vi "NMR13.vi"() -> ()   [LabVIEW 2013]
uses:
  <vilib>/Analysis/NI_AALBase.lvlib
panel:
  in  "AutoBaseline":bool=TRUE
  out "RF OK":bool=TRUE
  out "Peak area (V-MHz)":sgl=0.08843879 format="%.3f"
  in  "Gauss Fit":bool
  out "NMR Graph + Fit":cluster{cluster{dbl, "Numeric":dbl}[]}[](graph)=[{[{212.6, "Numeric"=0.037403535286502254}, {212.608, "Numeric"=0.009076660286615634}, {212.61599999999999, "Numeric"=0.027280678255148183}, {212.624, "Numeric"=0.041539514974009595}, {212.632, "Numeric"=0.042392721224115915}, {212.64, "Numeric"=0.02815572669266192}, {212.648, "Numeric"=0.028369547005266005}, {212.656, "Numeric"=0.02612744388036531}, {212.664, "Numeric"=0.028228733723923927}, {212.672, "Numeric"=0.03396540872402104}, {212.68, "Numeric"=0.032192449349113195}, {212.688, "Numeric"=0.03708221888018509}, {212.696, "Numeric"=0.032277295442774745}, {212.704, "Numeric"=0.033878753255359884}, {212.712, "Numeric"=0.03956725638019448}, {212.72, "Numeric"=0.02444046106777714}, {212.728, "Numeric"=0.03311506653637314}, {212.736, "Numeric"=0.03391382669270321}, {212.744, "Numeric"=0.028289378255278386}, {212.752, "Numeric"=0.03139064700513733}, {212.76, "Numeric"=0.034697125130210116}, {212.768, "Numeric"=0.022986644661528388}, {212.776, "Numeric"=0.0246283462239002}, {212.784, "Numeric"=0.020225257161465893}, {212.792, "Numeric"=0.019823764192777038}, {212.79999999999998, "Numeric"=0.024168496223911762}, {212.808, "Numeric"=0.019062675911470317}, {212.816, "Numeric"=0.019752885286524247}, {212.82399999999998, "Numeric"=0.015045276692672138}, {212.832, "Numeric"=0.0044881899739736}, {212.84, "Numeric"=0.013533285286520313}, {212.84799999999998, "Numeric"=0.028093648567681206}, {212.856, "Numeric"=0.011194182161475441}, {212.864, "Numeric"=0.04047160481776502}, {212.87199999999999, "Numeric"=0.029683240755188967}, {212.88, "Numeric"=0.03155125794272601}, {212.888, "Numeric"=0.01863425013025849}, {212.896, "Numeric"=0.03868612356769546}, {212.904, "Numeric"=0.05375521809897532}, {212.912, "Numeric"=0.05373411184900062}, {212.92, "Numeric"=0.0648435079427006}, {212.928, "Numeric"=0.08718106263022335}, {212.936, "Numeric"=0.10025117044274146}, {212.944, "Numeric"=0.1585216048177045}, {212.952, "Numeric"=0.2650075024739701}, {212.96, "Numeric"=0.46508239856773104}, {212.968, "Numeric"=0.8254088907552071}, {212.976, "Numeric"=1.0513580727864655}, {212.984, "Numeric"=0.8573220345052025}, {212.992, "Numeric"=0.6793237251302083}, {213.0, "Numeric"=0.6370530860677096}, {213.008, "Numeric"=0.6190965430989597}, {213.016, "Numeric"=0.49919677200520834}, {213.024, "Numeric"=0.44351588216145243}, {213.032, "Numeric"=0.4586334634114655}, {213.04, "Numeric"=0.47208857825520706}, {213.048, "Numeric"=0.434772339973944}, {213.056, "Numeric"=0.4489796704427201}, {213.064, "Numeric"=0.46391711263020446}, {213.072, "Numeric"=0.3840036118489343}, {213.08, "Numeric"=0.27875821106772336}, {213.088, "Numeric"=0.2001462423177006}, {213.096, "Numeric"=0.12634153372392326}, {213.104, "Numeric"=0.10264437825522532}, {213.112, "Numeric"=0.09343465872394546}, {213.12, "Numeric"=0.0575136446614109}, {213.12800000000001, "Numeric"=0.03758153138022602}, {213.136, "Numeric"=0.021797498567688922}, {213.144, "Numeric"=-0.00047077799485278904}, {213.15200000000002, "Numeric"=-0.0034786694010245367}, {213.16, "Numeric"=0.020452047005181218}, {213.168, "Numeric"=0.045967367317632346}, {213.17600000000002, "Numeric"=0.0187704165364736}, {213.184, "Numeric"=-0.008209117838577862}, {213.192, "Numeric"=-0.014756392057383827}, {213.2, "Numeric"=-0.02673810533852966}, {213.208, "Numeric"=-0.04046773424483824}, {213.216, "Numeric"=-0.046704556119901375}, {213.224, "Numeric"=-0.05625179361978411}, {213.232, "Numeric"=-0.04296198580734978}, {213.24, "Numeric"=-0.05743327721347158}, {213.248, "Numeric"=-0.06834242565103987}, {213.256, "Numeric"=-0.06423923580736263}, {213.264, "Numeric"=-0.06864665690097155}, {213.272, "Numeric"=-0.07023656393229688}, {213.28, "Numeric"=-0.056496749869876794}, {213.288, "Numeric"=-0.045896452994722836}, {213.296, "Numeric"=-0.05285217721355545}, {213.304, "Numeric"=-0.03777652018239258}, {213.312, "Numeric"=-0.024912645963475255}, {213.32, "Numeric"=-0.030617976432314953}, {213.328, "Numeric"=-0.02721917174490912}, {213.336, "Numeric"=-0.029767501432229004}, {213.344, "Numeric"=-0.01918337565107603}, {213.352, "Numeric"=-0.013301267057427346}, {213.36, "Numeric"=-0.01544148815098395}, {213.368, "Numeric"=-0.004363804557338036}, {213.376, "Numeric"=0.001474752473802965}, {213.38400000000001, "Numeric"=0.00859273763025964}, {213.392, "Numeric"=0.012363686067648316}, {213.4, "Numeric"=0.002082031380032434}]}]
  in  "Amp of Q curve":dbl=14.8 format="%_3f"
  in  "Subtract Q curve":bool=TRUE
  in  "Adjust Tune":bool
  out "IF Offset":dbl(graph)=3.0267583007812493
  out "Pedestal Difference":dbl(graph)=-0.055571065625063976
  out "# Good Spectra":i32=99
  in  "Quality cuts":bool=TRUE
  out "Pedestal OK":bool=TRUE
  out "Sweep #":i32=100
  out "1st Sweep":bool
  out "ADC volts OK":bool=TRUE
  out "Peak Height Distribution":cluster{"Y":dbl[], "Y":dbl[]}[](graph)=[{"Y"=[1.0290775755533925, 1.0294921670247466, 1.0299067584961008, 1.030321349967455, 1.030735941438809, 1.0311505329101633, 1.0315651243815174, 1.0319797158528716, 1.0323943073242259, 1.03280889879558, 1.0332234902669342, 1.0336380817382884, 1.0340526732096424, 1.0344672646809967, 1.0348818561523507, 1.035296447623705, 1.0357110390950592, 1.0361256305664133, 1.0365402220377675, 1.0369548135091216, 1.0373694049804758, 1.03778399645183, 1.038198587923184, 1.0386131793945383, 1.0390277708658924, 1.0394423623372466, 1.0398569538086009, 1.040271545279955, 1.0406861367513092, 1.0411007282226632, 1.0415153196940174, 1.0419299111653717, 1.0423445026367257, 1.04275909410808, 1.0431736855794342, 1.0435882770507883, 1.0440028685221425, 1.0444174599934966, 1.0448320514648508, 1.045246642936205, 1.045661234407559, 1.0460758258789133, 1.0464904173502674, 1.0469050088216216, 1.0473196002929759, 1.04773419176433, 1.0481487832356842, 1.0485633747070382, 1.0489779661783925, 1.0493925576497467, 1.0498071491211007, 1.050221740592455, 1.0506363320638092, 1.0510509235351633, 1.0514655150065175, 1.0518801064778716, 1.0522946979492258, 1.05270928942058, 1.053123880891934, 1.0535384723632883, 1.0539530638346424, 1.0543676553059966, 1.0547822467773509, 1.055196838248705, 1.0556114297200592, 1.0560260211914132, 1.0564406126627675, 1.0568552041341217, 1.0572697956054757, 1.05768438707683, 1.058098978548184, 1.0585135700195383, 1.0589281614908925, 1.0593427529622466, 1.0597573444336008, 1.060171935904955, 1.060586527376309, 1.0610011188476633, 1.0614157103190174, 1.0618303017903716, 1.0622448932617259, 1.06265948473308, 1.0630740762044342, 1.0634886676757882, 1.0639032591471425, 1.0643178506184967, 1.0647324420898507, 1.065147033561205, 1.065561625032559, 1.0659762165039133, 1.0663908079752675, 1.0668053994466216, 1.0672199909179758, 1.06763458238933, 1.068049173860684, 1.0684637653320384, 1.0688783568033924, 1.0692929482747466, 1.0697075397461009, 1.070122131217455], "Y"=[1.0, 0.0, 0.0, 0.0, 0.0, 0.0, 0.0, 0.0, 0.0, 0.0, 0.0, 0.0, 0.0, 1.0, 0.0, 0.0, 0.0, 0.0, 0.0, 1.0, 1.0, 0.0, 0.0, 2.0, 0.0, 0.0, 0.0, 2.0, 0.0, 2.0, 0.0, 2.0, 0.0, 3.0, 0.0, 4.0, 2.0, 1.0, 1.0, 2.0, 1.0, 1.0, 2.0, 0.0, 0.0, 2.0, 0.0, 1.0, 1.0, 1.0, 1.0, 2.0, 1.0, 3.0, 2.0, 1.0, 0.0, 4.0, 2.0, 1.0, 3.0, 1.0, 1.0, 4.0, 3.0, 3.0, 2.0, 0.0, 2.0, 0.0, 2.0, 0.0, 1.0, 2.0, 1.0, 1.0, 2.0, 3.0, 1.0, 1.0, 0.0, 1.0, 0.0, 1.0, 2.0, 0.0, 0.0, 1.0, 1.0, 2.0, 1.0, 1.0, 2.0, 0.0, 0.0, 1.0, 0.0, 1.0, 0.0, 1.0]}]
  in  "# of Sweeps":i32=100
  out "Std Dev (V)":dbl=0.008821657917615048 format="%_2g"
  out "Peak mean (V)":dbl=1.0528182762205458 format="%_4g"
  out "Peak Height":dbl(graph)=1.0513580727864655
  in  "Raw Data":bool=TRUE
  in  "Tank RF ON":bool=TRUE
  in  "IF Atten (dB)":i8 min=0 max=35 step=5
  in  "IFoffset (V)":dbl=3.026265771484374 min=0.0 max=3000.0 step=0.001 format="%.3f"
  in  "Tune  (V)":dbl=1.9290000000000005 min=0.0 max=5.0 step=0.001 format="%.3f"
  in  "Hi / Lo Gain":bool
  out "Voltage Array":sgl[](array[numeric])=[2.0380492, 1.9150025, 1.8403809, 1.7637085, 1.675525, 1.5741456, 1.4891113, 1.4035156, 1.3241577, 1.2503296, 1.1708863, 1.1, 1.0213134, 0.95092773, 0.8865234, 0.8031982, 0.7455689, 0.681958, 0.61381835, 0.55629885, 0.50087893, 0.43233642, 0.37904054, 0.32159424, 0.27004394, 0.22513428, 0.17266846, 0.12789306, 0.07961426, 0.027380371, -0.0033569336, -0.026684571, -0.07957764, -0.08439942, -0.12739258, -0.15583496, -0.19716796, -0.20363769, -0.2131958, -0.23594971, -0.24567871, -0.24228516, -0.24626465, -0.20314941, -0.10992432, 0.07878418, 0.42963868, 0.64801025, 0.448291, 0.2665039, 0.22233887, 0.20438233, 0.08637695, 0.034484863, 0.055285644, 0.07631836, 0.04847412, 0.07404785, 0.10224609, 0.037487794, -0.050708007, -0.11037598, -0.16334228, -0.16430664, -0.14888915, -0.15828857, -0.14980468, -0.13527831, -0.1253418, -0.094250485, -0.034326173, 0.029077148, 0.041662596, 0.056359865, 0.09338379, 0.12686768, 0.16049805, 0.20351562, 0.24511719, 0.31145018, 0.3519165, 0.39783937, 0.46066895, 0.5168823, 0.5778076, 0.65595704, 0.73286134, 0.794104, 0.87927246, 0.96412355, 1.0322998, 1.1114746, 1.1865966, 1.2767456, 1.3640869, 1.4453003, 1.541626, 1.634607, 1.7307618, 1.8254639, 1.9080079] format="%.4f"
  in  "Invert Polarity":bool=TRUE
  out "Pedestal Diff (V)":sgl=-0.055571064 format="%.3f"
  out "Peak amp (V)":sgl=1.0513581 format="%.3f"
  in  "Save Data to File":bool
  in  "RF Level (dBm)":dbl min=-10.0 max=1.0 step=0.1 format="%.2f"
  out "SMT error out":errorcluster
  out "Sample RMS (V)":dbl=0.013290809562570826 format="%.4f"
  in  "# Sample/step":i32=100 min=1 max=1000 step=100
  in  "ADC Rate (Hz)":i32=10000 min=1 max=20000 step=1000
  in  "ADC Range":i32(ring)=1 items=["+- 10 V"=1, "+- 2.5 V"=3]
  in  "Step Width (MHz)":dbl=0.008 min=0.0 max=1000.0 step=0.0005 format="%.4f"
  in  "Freq Span (MHz)":dbl=0.8 min=0.0 max=3000.0 step=0.1 format="%.3f"
  in  "Center Freq (MHz)":dbl=213.0 min=0.005 max=6000.0 step=0.1 format="%.3f"
  in  "Sweep Mode":u16(ring)=3 items=["Off", "Single", "Auto", "Step"]
  in  "GPIB Addr (28)":refnum<visa-resource-name>="GPIB0::28::INSTR"
  # "Settings"
  # "E1039 Prototype NMR Control Panel"
  # "D\nA\nC"
  # "R\nF\n\nG\ne\nn\ne\nr\na\nt\no\nr"
  # "A\nD\nC"
  # "D\na\nt\na"
  # "I\n/\nO"
  # "Results"
  # "A\nv\ne\nr\na\ng\ne"
  # "S\nw\ne\ne\np"
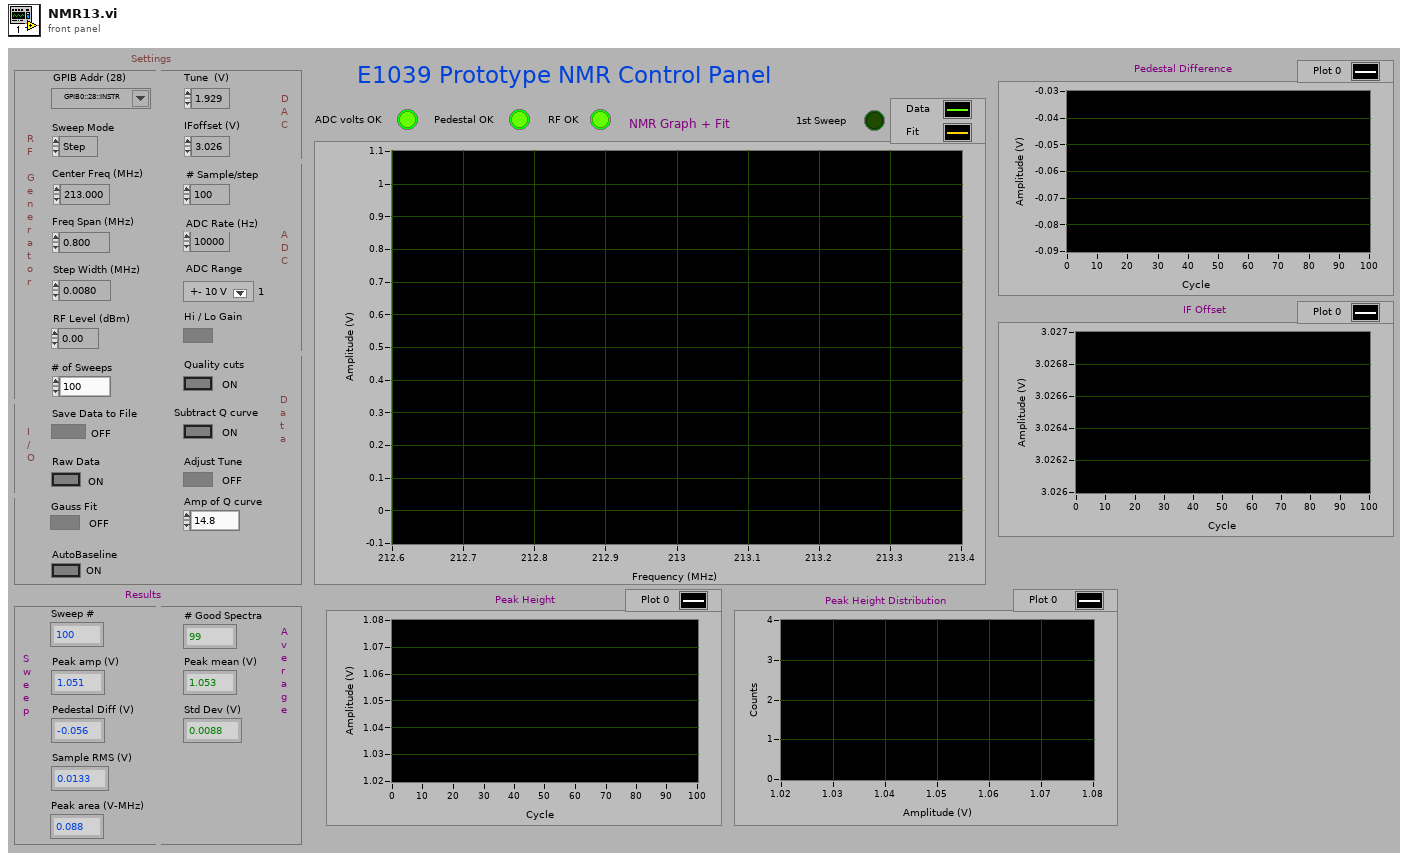
[diagram p1: front panel]
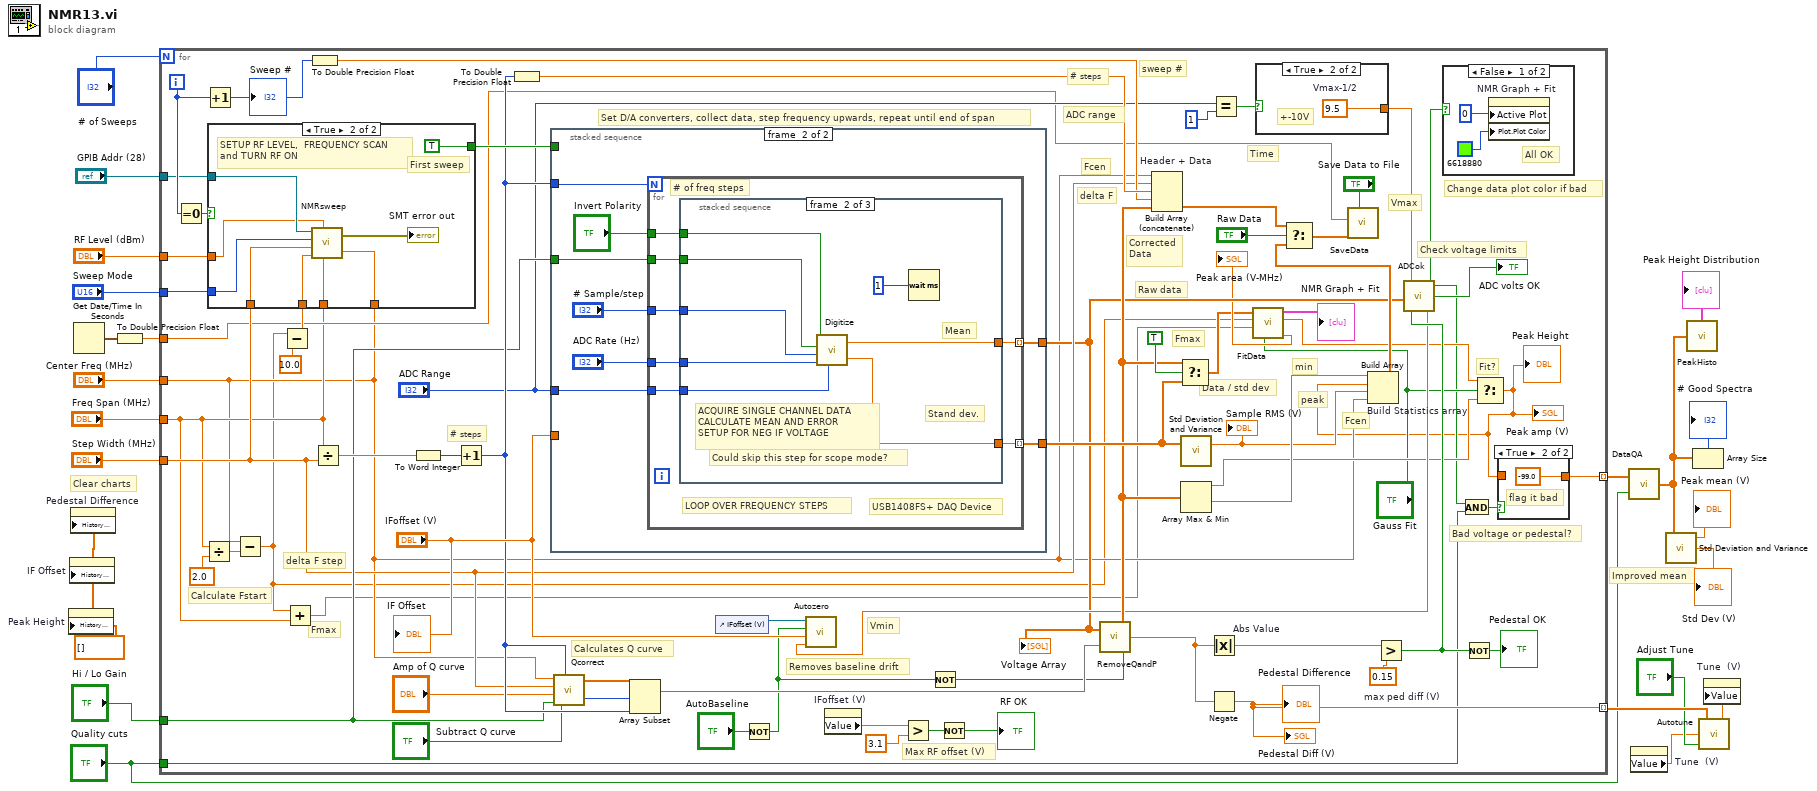
[diagram p0: block diagram]
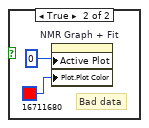
[diagram p2: hidden frame]
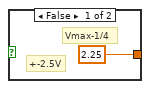
[diagram p3: hidden frame]
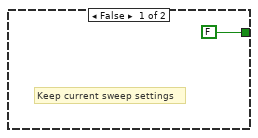
[diagram p5: hidden frame]
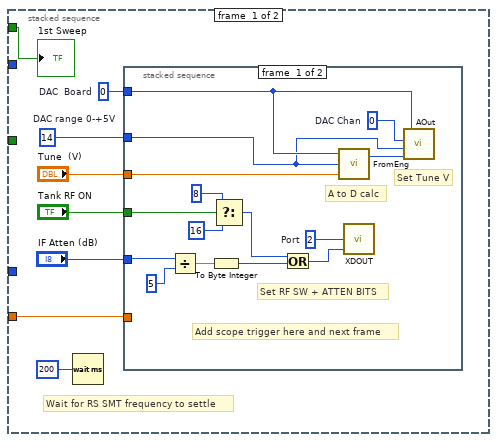
[diagram p6: hidden frame]
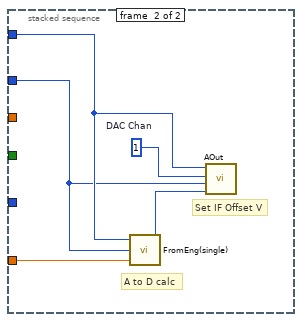
[diagram p7: hidden frame]
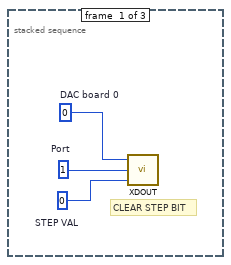
[diagram p8: hidden frame]
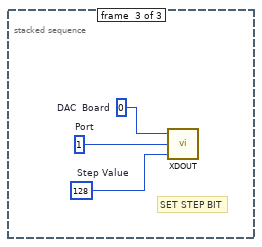
[diagram p9: hidden frame]
diagram:
  w6 = dbl[] []
  # "Clear charts"
  # "Improved mean"
  n1 = property on="Peak Height" class="WFChart (strict)"("History Data"=w6) -> ()  [unwired: 2 in, 2 out]
  n2 = property on="IF Offset" class="WFChart (strict)"("History Data"=w6) -> ()  [unwired: 2 in, 2 out]
  n3 = property on="Pedestal Difference" class="WFChart (strict)"("History Data"=w6) -> ()  [unwired: 2 in, 2 out]
  n4 = Get Date/Time In Seconds() -> (seconds since 1Jan1904=w2:timestamp)
  n5 = To Double Precision Float(number=w2) -> (double precision float=w1:dbl)
  n6 = for {
    N: "# of Sweeps" -> [_]
    tunnel: [w76] -> w18 mode=indexing
    tunnel: "Quality cuts" -> [w48]
    tunnel: [w57] -> w15 mode=indexing
    tunnel: "Center Freq (MHz)" -> [w35]
    tunnel: "Freq Span (MHz)" -> [w41]
    tunnel: "Step Width (MHz)" -> [w47]
    tunnel: "Sweep Mode" -> [w61]
    tunnel: "Hi / Lo Gain" -> [w60]
    tunnel: "GPIB Addr (28)" -> [w59]
    tunnel: "RF Level (dBm)" -> [w58]
    tunnel: w1 -> [w42]
    i -> [w74]
    w77 = 0.15  # max ped diff (V)
    # "Vmax"
    # "Change data plot color if bad"
    # "Max RF offset (V)"
    # "Fmax"
    # "Fit?"
    # "Fmax"
    # "Time"
    # "Vmin"
    # "min"
    # "peak"
    # "Raw data"
    # "Corrected\nData"
    # "Fcen"
    # "delta F"
    # "# steps"
    # "ADC range"
    # "sweep #"
    # "Fcen"
    # "Set D/A converters, collect data, step frequency upwards, repeat until end of span"
    # "Calculates Q curve"
    # "Removes baseline drift"
    # "Bad voltage or pedestal?"
    # "Check voltage limits"
    # "Data / std dev"
    # "# steps"
    # "Calculate Fstart"
    # "delta F step"
    n7 = Equal To 0?(x=w74) -> (x = 0?=w79:bool)
    n8 = Divide(x=w41, y=sgl 2.0) -> (x/y=w91:dbl)
    n9 = Increment(x=w74) -> (x+1=w64:i32)
    "Sweep #" <- w64
    n10 = Subtract(x=w35, y=w91) -> (x-y=w30:dbl)
    n11 = Subtract(x=w30, y=10.0) -> (x-y=w89:dbl)
    n12 = case shown="True" w79 {
      tunnel: w89 -> [_ w111]
      tunnel: w47 -> [_ w109]
      tunnel: w35 -> [_ w108]
      tunnel: w41 -> [_ w110]
      tunnel: [FALSE TRUE] -> w78
      tunnel: w61 -> [_ w105]
      tunnel: w59 -> [_ w104]
      tunnel: w58 -> [_ w103]
      frame False {
        # "Keep current sweep settings"
      }
      frame True {
        # "First sweep"
        # "SETUP RF LEVEL,  FREQUENCY SCAN\nand TURN RF ON"
        n13 = call "NMRsweep.vi"("Center Freq (MHz)"=w108, "Freq Span (MHz)"=w110, "RF Level (dBm)"=w103, "Foffset (MHz)"=w111, "Step Width (MHz)"=w109, "Sweep Mode"=w105, "GPIB Addr (28)"=w104) -> ("error out"=→"SMT error out":errorcluster)
      }
    }
    n14 = Add(x=w30, y=w41) -> (x+y=w29:dbl)
    n15 = To Double Precision Float(number=w64) -> (double precision float=w65:dbl)
    n16 = Divide(x=w41, y=w47) -> (x/y=w93:dbl)
    n17 = To Word Integer(number=w93) -> (16bit integer=w90:i16)
    n18 = Increment(x=w90) -> (x+1=w68:i16)
    n19 = To Double Precision Float(number=w68) -> (double precision float=w67:dbl)
    n20 = stacked-sequence {
      tunnel: [_ w147] -> w82
      tunnel: [_ w146] -> w45
      tunnel: w68 -> [_ w145]
      tunnel: "IFoffset (V)" -> [w113 _]
      tunnel: w60 -> [_ w144]
      tunnel: w78 -> [w112 _]
      tunnel: "ADC Range" -> [_ w143]
      frame #0 {
        w117 = 14  # DAC range 0-+5V
        w118 = 0  # DAC  Board
        # "Wait for RS SMT frequency to settle"
        n21 = Wait (ms)(milliseconds to wait=200) -> ()  [unwired: 1 out]
        n22 = stacked-sequence {
          tunnel: w118 -> [w125 w137]
          tunnel: w117 -> [w124 w136]
          tunnel: "Tune  (V)" -> [w123 _]
          tunnel: "Tank RF ON" -> [w121 _]
          tunnel: "IF Atten (dB)" -> [w120 _]
          tunnel: w113 -> [_ w135]
          frame #0 {
            w127 = 2  # Port
            w134 = 0  # DAC Chan
            # "Add scope trigger here and next frame"
            # "A to D calc"
            # "Set RF SW + ATTEN BITS"
            # "Set Tune V"
            n23 = Divide(x=w120, y=5) -> (x/y=w132:dbl)
            n24 = To Byte Integer(number=w132) -> (8bit integer=w129:i8)
            n25 = Select(t=8, s=w121, f=16) -> (s? t:f=w128:i32)
            n26 = Or(x=w128, y=w129) -> (x .or. y?=w126:i32)
            n27 = call-poly "FromEng.VI"("Eng Units"=w123, "Range"=w124, "BoardNum (0)"=w125) -> ("DA Data"=w122:u16)  [unwired: 1 out]
            n28 = call "XDOUT.VI"(2:w126, "PortNum"=w127) -> ()  [unwired: 3 in]
            n29 = call "AOut.VI"("DataValue"=w122, "Range"=w124, "Channel"=w134, "BoardNum"=w125) -> ()  [unwired: 1 out]
          }
          frame #1 {
            w139 = 1  # DAC Chan
            # "A to D calc"
            # "Set IF Offset V"
            n30 = call "FromEng(single).VI"("Eng Units"=w135, "Range"=w136, "BoardNum (0)"=w137) -> ("DA Data"=w138:u16)  [unwired: 1 out]
            n31 = call "AOut.VI"("DataValue"=w138, "Range"=w136, "Channel"=w139, "BoardNum"=w137) -> ()  [unwired: 1 out]
          }
        }
        "1st Sweep" <- w112
      }
      frame #1 {
        n32 = for {
          N: w145 -> [_]
          tunnel: [w154] -> w146 mode=indexing
          tunnel: [w153] -> w147 mode=indexing
          tunnel: w144 -> [w152]
          tunnel: w143 -> [w151]
          tunnel: "ADC Rate (Hz)" -> [w150]
          tunnel: "# Sample/step" -> [w149]
          tunnel: "Invert Polarity" -> [w148]
          # "# of freq steps"
          # "USB1408FS+ DAQ Device"
          # "LOOP OVER FREQUENCY STEPS"
          n33 = stacked-sequence {
            tunnel: [_ w164 _] -> w154
            tunnel: [_ w163 _] -> w153
            tunnel: w152 -> [_ w162 _]
            tunnel: w151 -> [_ w161 _]
            tunnel: w150 -> [_ w160 _]
            tunnel: w149 -> [_ w159 _]
            tunnel: w148 -> [_ w158 _]
            frame #0 {
              w155 = 0  # DAC board 0
              w156 = 0  # STEP VAL
              w157 = 1  # Port
              # "CLEAR STEP BIT"
              n34 = call "XDOUT.VI"(2:w156, "PortNum"=w157, "BoardNum"=w155) -> ()  [unwired: 2 in]
            }
            frame #1 {
              # "Could skip this step for scope mode?"
              # "Stand dev."
              # "Mean"
              # "ACQUIRE SINGLE CHANNEL DATA\nCALCULATE MEAN AND ERROR\nSETUP FOR NEG IF VOLTAGE"
              n35 = call "Digitize.vi"("Invert Polarity"=w158, "IF or Log"=w162, "# Sample/step"=w159, "ADC Rate (Hz)"=w160, "ADC Range"=w161) -> ("mean"=w164:dbl, "standard deviation"=w163:dbl)
              n36 = Wait (ms)(milliseconds to wait=1) -> ()  [unwired: 1 out]
            }
            frame #2 {
              w166 = 128  # Step Value
              w168 = 0  # DAC  Board
              w167 = 1  # Port
              # "SET STEP BIT"
              n37 = call "XDOUT.VI"(2:w166, "PortNum"=w167, "BoardNum"=w168) -> ()  [unwired: 2 in]
            }
          }
        }
      }
    }
    "Voltage Array" <- w45
    n38 = call "Qcorrect.vi"("Subtract Q curve"="Subtract Q curve", "Nstep"=w68, "IF or Log"=w60, "Amp of Q curve"="Amp of Q curve", "Step Width (MHz)"=w47, "Center Freq (MHz)"=w35) -> ("Start"=w84:i32, "Array"=w85:dbl[])
    n39 = Array Subset "Array Subset"(array=w85, index=w84, length=w68) -> (w83:dbl[])
    n40 = control-ref of="IFoffset (V)"() -> (w51:refnum<vi>)
    n41 = Not(x="AutoBaseline") -> (.not. x?=w24:bool)
    n42 = property on="IFoffset (V)" class="DigNum (strict)"() -> ("Value"=w39:dbl)  [unwired: 2 in, 2 out]
    n43 = Greater?(x=w39, y=3.1) -> (0:w37:bool)
    n44 = Not(x=w24) -> (.not. x?=w23:bool)
    n45 = Not(x=w37) -> (.not. x?=→"RF OK":bool)
    n46 = call "RemoveQandP.vi"("Raw data"=w45, "Qcurve"=w83, "Subtract Ped?"=w23) -> ("Corrected data"=w66:dbl[], "Ped L-R"=w70:dbl)
    n47 = Build Array (concatenate) "Header + Data"(w35, w47, w67, w65, w66) -> (w69:dbl[])
    n48 = Select(t=w66, s=TRUE, f=w82) -> (s? t:f=w31:dbl[])
    n49 = call <vilib>:"Std Deviation and Variance.vi"("X"=w82) -> ("mean"=w46:dbl)  [unwired: 1 in, 2 out]
    "Sample RMS (V)" <- w46
    n50 = Array Max & Min(array=w66) -> (max value=w40:dbl, min value=w81:dbl)  [unwired: 2 out]
    n51 = Absolute Value "Abs Value"(x=w70) -> (abs(x)=w72:dbl)
    n52 = Negate(x=w70) -> (-x=w57:dbl)
    "Pedestal Diff (V)" <- w57
    "Pedestal Difference" <- w57
    n53 = Equal?(x="ADC Range", y=1) -> (x = y?=w55:bool)
    n54 = call "FitData.vi"("Fit?"="Gauss Fit", "Fmax"=w29, "Fmin"=w30, "Yarray"=w31) -> ("Peak Area (V-MHz)"=→"Peak area (V-MHz)":dbl, "Amplitude (V)"=w33:dbl, "NMR Graph + Fit"=→"NMR Graph + Fit":cluster{cluster{dbl, "Numeric":dbl}[]}[])  [unwired: 2 out]
    n55 = case shown="True" w55 {
      tunnel: [2.25 w99] -> w52
      frame False {
        # "Vmax-1/4"
        # "+-2.5V"
      }
      frame True {
        w99 = 9.5  # Vmax-1/2
        # "+-10V"
      }
    }
    n56 = Greater?(x=w72, y=w77) -> (0:w56:bool)
    n57 = call "ADCok.vi"("PedOK"=w56, "Array"=w45, "Vmax-1/2"=w52) -> ("Vmin"=w50:dbl, "ADC voltages OK"=→"ADC volts OK":bool, "Allok"=w27:bool)
    n58 = call "Autozero.vi"("Vmin (V)"=w50, "IFoffset (V)"="IFoffset (V)", "IF or Log"=w24, "reference"=w51) -> ()
    n59 = case shown="False" w27 {
      frame False {
        # "All OK"
        n60 = property on="NMR Graph + Fit" class="XYGraph (strict)"("Active Plot"=0, "Plot.Plot Color"=u32 6618880) -> ()  [unwired: 2 in, 2 out]
      }
      frame True {
        # "Bad data"
        n61 = property on="NMR Graph + Fit" class="XYGraph (strict)"("Active Plot"=0, "Plot.Plot Color"=u32 16711680) -> ()  [unwired: 2 in, 2 out]
      }
    }
    n62 = And(x=w27, y=w48) -> (x .and. y?=w73:bool)
    n63 = Not(x=w56) -> (.not. x?=→"Pedestal OK":bool)
    n64 = Select(t=w33, s="Gauss Fit", f=w40) -> (s? t:f=w26:dbl)
    "Peak amp (V)" <- w26
    "Peak Height" <- w26
    n65 = Build Array "Build Statistics array"(w81, w26, w46, w35) -> (w88:dbl[])
    n66 = Select(t=w69, s="Raw Data", f=w88) -> (s? t:f=w43:dbl[])
    n67 = call "SaveData.vi"("Array"=w43, "Save Data to File"="Save Data to File", "Ext time (sec)"=w42) -> ()  [unwired: 1 out]
    n68 = case shown="True" w73 {
      tunnel: [w100 -99.0] -> w76
      tunnel: w26 -> [w100 _]
      frame False {
        # "Data OK"
      }
      frame True {
        # "flag it bad"
      }
    }
    "IF Offset" <- "IFoffset (V)"
  }
  n69 = call "DataQA.vi"("Quality cuts"="Quality cuts", "Data In"=w18) -> ("Data Out"=w17:dbl[])
  n70 = property on="Tune  (V)" class="DigNum (strict)"() -> ("Value"=w5:dbl)  [unwired: 2 in, 2 out]
  n71 = call <vilib>:"Std Deviation and Variance.vi"("X"=w17) -> ("mean"=→"Peak mean (V)":dbl, "standard deviation"=→"Std Dev (V)":dbl)  [unwired: 1 in, 1 out]
  n72 = call "PeakHisto.vi"("Data Out"=w17) -> ("XY Graph"=→"Peak Height Distribution":cluster{"Y":dbl[], "Y":dbl[]}[])
  n73 = Array Size(array=w17) -> (size(s)=→"# Good Spectra":i32)
  n74 = call "Autotune.vi"("Adjust Tune"="Adjust Tune", "Tune Vin"=w5, "Pedestal Diff"=w15) -> ("Tune Vout"=w4:dbl)
  n75 = property on="Tune  (V)" class="DigNum (strict)"("Value"=w4) -> ()  [unwired: 2 in, 2 out]
